vi "最大值.vi"(10 "y":dbl, 11 "x":dbl) -> (3 "result":dbl)   [LabVIEW 2013]
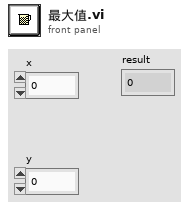
[diagram p1: front panel]
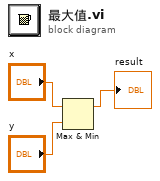
[diagram p0: block diagram]
diagram:
  n1 = Max & Min(x="x", y="y") -> (max(x,y)=→"result":dbl)  [unwired: 1 out]
